vi "S30c_dll F95.vi"(4 "error in":errorcluster, 5 "Comand":T1(ring), 7 "Dev Addr":u8=250) -> (0 "error out":errorcluster)   [LabVIEW 2014, in "K_S30c_dll.lvlib"]
uses:
  K_S30c_dll.lvlib
  s30c.dll
panel:
  # "Function 95: Set Zero\n\nusing s30c.dll\nKeller AG für Druckmesstechnik, 29.5.08 b.v."
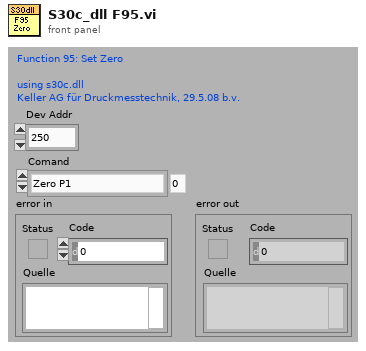
[diagram p1: front panel]
types:
  T1 = enum16{"Zero P1", "Set default zero of P1", "Zero P2", "Set defalut zero of P2", "not used", "not used_1", "Zero CH0", "Set defalut zero of CH0"}
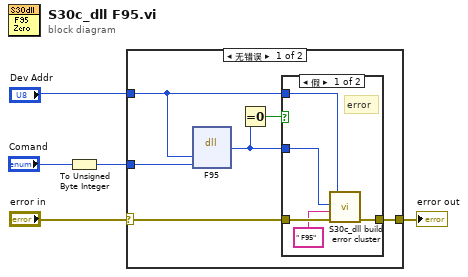
[diagram p0: block diagram]
diagram:
  n1 = To Unsigned Byte Integer(number="Comand") -> (unsigned 8bit integer=w2:u8)
  n2 = case shown="无错误" "error in" {
    selector: "error in" -> [w9 w18]
    tunnel: [w10 w18] -> w5
    tunnel: "Dev Addr" -> [w7 _]
    tunnel: w2 -> [w8 _]
    frame No Error {
      n3 = dll-call lib="PTH2Labs EworkSINOPEC北控自动相渗software2.08.5_dlls30c.dll" fn="F95"("DevAddr"=w7, "command"=w8) -> (w6:i16)  [unwired: 5 in, 2 out]
      n4 = Equal To 0?(x=w6) -> (x = 0?=w11:bool)
      n5 = case shown="假" w11 {
        tunnel: [w15 w17] -> w10
        tunnel: w9 -> [w16 w17]
        tunnel: w7 -> [w13 _]
        tunnel: w6 -> [w12 _]
        frame False {
          # "error"
          n6 = call "S30c_dll build error cluster.vi"("error in"=w16, "error Text"=" F95", "error code"=w12, "Dev Addr"=w13) -> ("error out"=w15:errorcluster)  [unwired: 3 in]
        }
        frame True {
        }
      }
    }
    frame Error {
    }
  }
  "error out" <- w5
